vi "CountsToUnit.vi"(0 "Counts":i32, 1 "Target Units (default mm)":enum16{"mm", "µm"}(ring)) -> (2 "mm":dbl, 3 "target units value":dbl, 4 "µm":dbl)   [LabVIEW 2023]
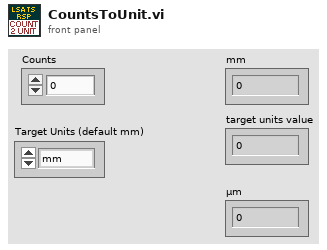
[diagram p1: front panel]
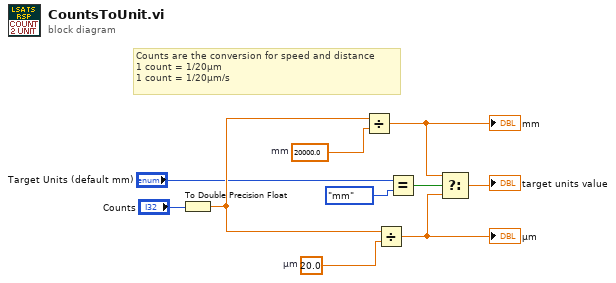
[diagram p0: block diagram]
diagram:
  w9 = 20.0  # µm
  w10 = 20000.0  # mm
  # "Counts are the conversion for speed and distance \n1 count = 1/20µm\n1 count = 1/20µm/s"
  n1 = To Double Precision Float(number="Counts") -> (double precision float=w7:dbl)
  n2 = Divide(x=w7, y=w10) -> (x/y=w3:dbl)
  "mm" <- w3
  n3 = Divide(x=w7, y=w9) -> (x/y=w2:dbl)
  "µm" <- w2
  n4 = Equal?(x="Target Units (default mm)", y=enum16{"mm", "µm"}."mm" ("Target Units")) -> (x = y?=w6:bool)
  n5 = Select(t=w3, s=w6, f=w2) -> (s? t:f=→"target units value":dbl)
